vi "Rename.vi"(5 "Username":string, 6 "Password":string, 7 "Address":string, 8 "Error In":errorcluster) -> (0 "Error Out":errorcluster)   [LabVIEW 2018, in "Tests.lvlib" / "SFTP.lvlib"]
uses:
  SFTP.lvlib
  src/Toolkit/SFTP File/Type Definitions/Open Options.ctl
  src/Toolkit/SFTP/Support/Create from Session.vi
  src/Toolkit/SFTP File/Support/Open from SFTP.vi
  src/Toolkit/SFTP File/Support/Close to SFTP.vi
  src/Toolkit/SFTP/Support/Destroy to Session.vi
  <vilib>/addons/_JKI Toolkits/Caraya/classes/Test/Test.lvclass
  <vilib>/addons/_JKI Toolkits/Caraya/classes/Assert/Assert.lvclass
  src/Toolkit/SFTP/SFTP.lvclass
  src/Toolkit/SFTP File/SFTP File.lvclass
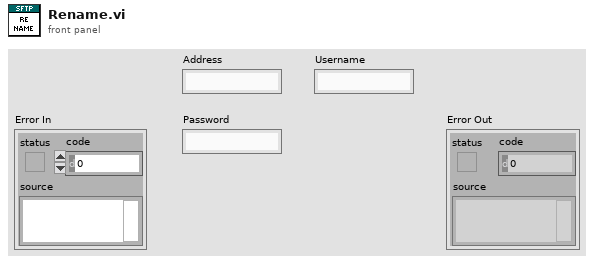
[diagram p1: front panel]
types:
  T1 = typedef "Toolkit.lvlib/SFTP File.lvclass/Open Options.ctl" = cluster{"Read":bool, "Write":bool, "Append":bool, "Create":bool, "Truncate":bool, "Exclude":bool}
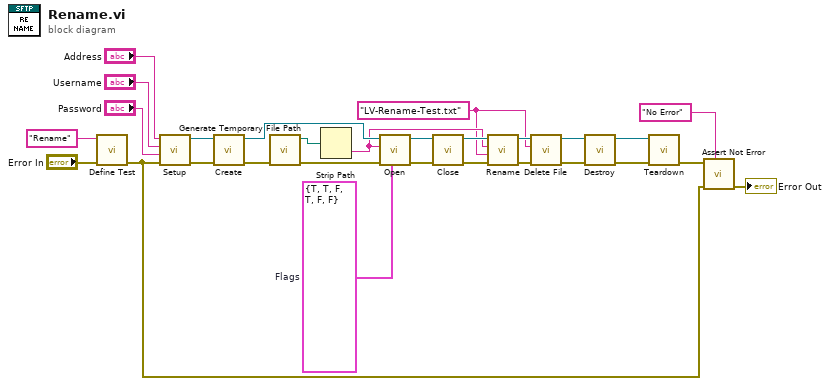
[diagram p0: block diagram]
diagram:
  w1 = "LV-Rename-Test.txt" ("Remote Destination Path")
  w13 = T1 {"Read"=TRUE, "Write"=TRUE, "Append"=FALSE, "Create"=TRUE, "Truncate"=FALSE, "Exclude"=FALSE}  # Flags
  n1 = call <vilib>:"Define Test.vi"("error in (no error)"="Error In", "Label (VI Title)"="Rename") -> ("error out"=w23:errorcluster)  [unwired: 9 in]
  n2 = call "Setup.vi"("Error In"=w23, "Password"="Password", "Username"="Username", "Address"="Address") -> ("Error Out"=w24:errorcluster, "Sesssion"=w19:refnum<class "Session.lvclass">)  [unwired: 6 in]
  n3 = call-poly "Create.vi"("Error In"=w24, "Session"=w19) -> ("Error Out"=w12:errorcluster, "SFTP"=w11:refnum<class "SFTP.lvclass">)  [unwired: 8 in]
  n4 = call <vilib>:"Generate Temporary File Path.vi"("error in (no error)"=w12) -> ("error out"=w15:errorcluster, "Unique Temporary File Path"=w14:path)  [unwired: 9 in]
  n5 = Strip Path(path=w14) -> (name=w6:string)  [unwired: 1 out]
  n6 = call-poly "Open.vi"("Options"=w13, "Error In"=w15, "Remote Path"=w6, "SFTP"=w11) -> ("Error Out"=w9:errorcluster, "SFTP File"=w10:refnum<class "SFTP File.lvclass">)  [unwired: 6 in]
  n7 = call-poly "Close.vi"("Error In"=w9, "SFTP File"=w10) -> ("Error Out"=w8:errorcluster, "SFTP"=w7:refnum<class "SFTP.lvclass">)  [unwired: 7 in, 1 out]
  n8 = call "Rename.vi"("Error In"=w8, "Remote Destination Path"=w1, "Remote Source Path"=w6, "SFTP In"=w7) -> ("Error Out"=w4:errorcluster, "SFTP Out"=w5:refnum<class "SFTP.lvclass">)  [unwired: 6 in]
  n9 = call "Delete File.vi"("Error In"=w4, "Remote Path"=w1, "SFTP In"=w5) -> ("Error Out"=w3:errorcluster, "SFTP Out"=w2:refnum<class "SFTP.lvclass">)  [unwired: 7 in]
  n10 = call-poly "Destroy.vi"("Error In"=w3, "SFTP"=w2) -> ("Error Out"=w18:errorcluster, "Session"=w16:refnum<class "Session.lvclass">)  [unwired: 8 in]
  n11 = call "Teardown.vi"("Error In"=w18, "Session"=w16) -> ("Error Out"=w17:errorcluster)  [unwired: 9 in]
  n12 = call <vilib>:"Assert Not Error.vi"("Label"="No Error", "error in (no error)"=w23, "Not Error?"=w17) -> ("error out"=→"Error Out":errorcluster)  [unwired: 8 in]
